vi "Rec Fetch Datetime Data (R).vi"(6 "error in (no error)":errorcluster, 7 "type":string, 8 "column index":variant, 9 "recordset reference":T1) -> (0 "error out":errorcluster, 1 "data":string, 3 "recordset reference out":T1)   [LabVIEW 2012, in "NI_Database_API_64.lvlib"]
doc: "Retrieves the data located at the <B>column index</B> of the current record in the recordset identified by the <B>recordset reference</B>. The <B>column index</B> can be either the zero-indexed position of the column in the recordset or the name of the column. Wire data to the <B>type</B> input to determine the polymorphic instance to use or manually select the instance."
uses:
  NI_Database_API_64.lvlib
  _DB Variant To Data/Database Variant To Data.xnode
  Rec ObjectReference.ctl
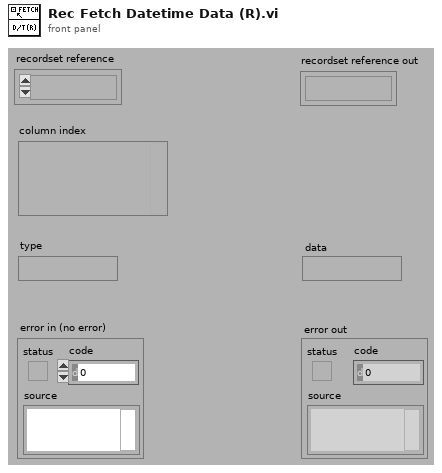
[diagram p1: front panel]
types:
  T1 = typedef "NI_Database_API_64.lvlib/Rec ObjectReference.ctl" = refnum<k1>
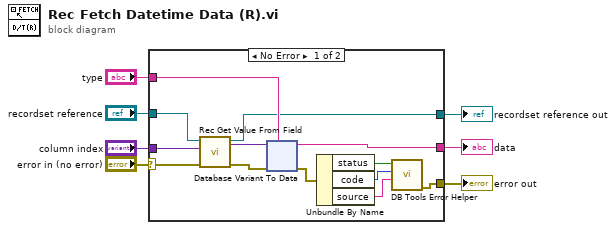
[diagram p0: block diagram]
diagram:
  n1 = case shown="No Error" "error in (no error)" {
    selector: "error in (no error)" -> [w8 w54]
    tunnel: "recordset reference" -> [w20 w53]
    tunnel: "type" -> [w18 _]
    tunnel: [w17 w53] -> w5
    tunnel: [w16 _] -> w4
    tunnel: "column index" -> [w15 _]
    tunnel: [w10 w54] -> w2
    frame No Error {
      n2 = call "Rec Get Value From Field.vi"("error in (no error)"=w8, "column index"=w15, "recordset reference"=w20) -> ("error out"=w19:errorcluster, "value"=w14:variant, "recordset reference out"=w17:T1)  [unwired: 1 in, 3 out]
      n3 = xnode "Database Variant To Data"("database variant"=w14, "error in"=w19, "type"=w18) -> ("data"=w16:string, "error out"=w11:errorcluster)
      n4 = Unbundle By Name(w11) -> ("status"=w12:bool, "code"=w9:i32, "source"=w13:string)
      n5 = call "DB Tools Error Helper.vi"("source"=w13, "code"=w9, "status"=w12) -> ("error out"=w10:errorcluster)  [unwired: 1 in, 7 out]
    }
    frame Error {
    }
  }
  "data" <- w4
  "error out" <- w2
  "recordset reference out" <- w5
